vi "设置电压.vi"(5 "布尔":bool, 8 "error out":errorcluster, 9 "V2设置值":i32, 10 "V1设置值":i32, 11 "VISA resource name out":refnum<visa-resource-name>) -> ()   [LabVIEW 2018]
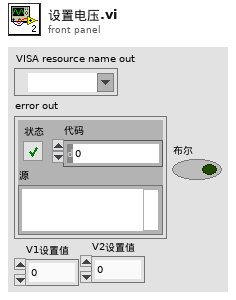
[diagram p1: front panel]
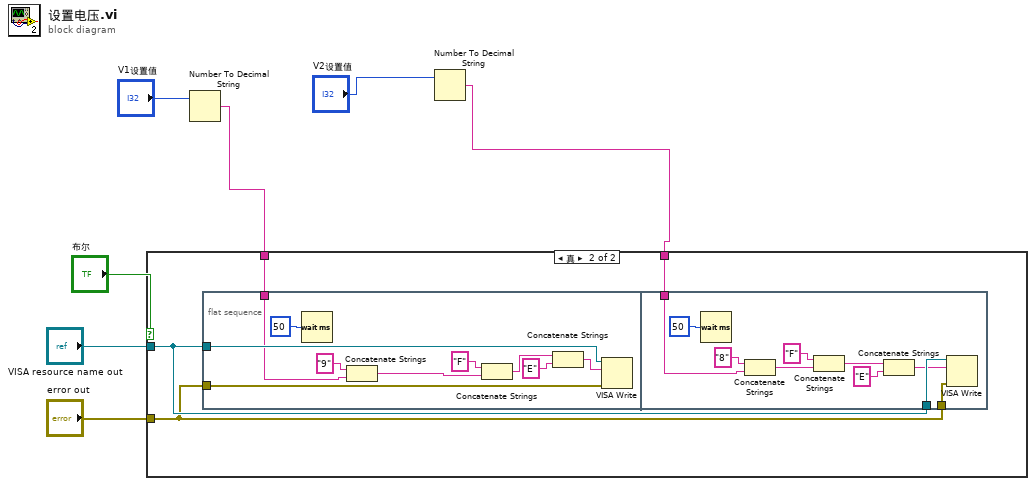
[diagram p0: block diagram]
diagram:
  n1 = Number To Decimal String(number="V1设置值") -> (decimal integer string=w3:string)  [unwired: 1 in]
  n2 = Number To Decimal String(number="V2设置值") -> (decimal integer string=w2:string)  [unwired: 1 in]
  n3 = case shown="真" "布尔" {
    tunnel: "VISA resource name out" -> [_ w11]
    tunnel: "error out" -> [_ w10]
    tunnel: w3 -> [_ w9]
    tunnel: w2 -> [_ w8]
    frame False {
    }
    frame True {
      n4 = flat-sequence {
        tunnel: w11 -> [w21]
        tunnel: w10 -> [w20]
        tunnel: w9 -> [w12]
        tunnel: w10 -> [w30]
        tunnel: w11 -> [w29]
        tunnel: w8 -> [w22]
        frame #0 {
          n5 = Wait (ms)(milliseconds to wait=50) -> ()  [unwired: 1 out]
          n6 = Concatenate Strings("9", w12) -> (w16:string)
          n7 = Concatenate Strings("F", w16) -> (w14:string)
          n8 = Concatenate Strings(w14, "E") -> (w13:string)
          n9 = VISA Write(VISA resource name=w21, write buffer=w13, error in (no error)=w20) -> ()  [unwired: 3 out]
        }
        frame #1 {
          n10 = Wait (ms)(milliseconds to wait=50) -> ()  [unwired: 1 out]
          n11 = Concatenate Strings("8", w22) -> (w25:string)
          n12 = Concatenate Strings("F", w25) -> (w26:string)
          n13 = Concatenate Strings(w26, "E") -> (w23:string)
          n14 = VISA Write(VISA resource name=w29, write buffer=w23, error in (no error)=w30) -> ()  [unwired: 3 out]
        }
      }
    }
  }
